vi "CIMAQ_ParticleFilter_MinMax.vi"(8 "error in (no error)":errorcluster, 9 "Max/Min":enum16{"Max", "Min"}(ring), 10 "Measurement Parameter":T1=35 items=["Center of Mass X", "Center of Mass Y", "First Pixel X", "First Pixel Y", "Bounding Rect Left", "Bounding Rect Top", "Bounding Rect Right", "Bounding Rect Bottom", "Max Feret Diameter Start X", "Max Feret Diameter Start Y", "Max Feret Diameter End X", "Max Feret Diameter End Y", "Max Horiz. Segment Length Left", "Max Horiz. Segment Length Right", "Max Horiz. Segment Length Row", "-", "Bounding Rect Width", "Bounding Rect Height", "Bounding Rect Diagonal", "Perimeter", "Convex Hull Perimeter", "Holes' Perimeter", "Max Feret Diameter", "Equivalent Ellipse Major Axis", "Equivalent Ellipse Minor Axis", "Equivalent Ellipse Minor Axis (Feret)", "Equivalent Rect Long Side", "Equivalent Rect Short Side", "Equivalent Rect Diagonal", "Equivalent Rect Short Side (Feret)", "Average Horiz. Segment Length", "Average Vert. Segment Length", "Hydraulic Radius", "Waddel Disk Diameter", "-", "Area", "Holes' Area", "Particle & Holes' Area", "Convex Hull Area", "Image Area", "-", "Number of Holes", "Number of Horiz. Segments", "Number of Vert. Segments", "-", "Orientation", "Max Feret Diameter Orientation", "-", "% Area/Image Area", "% Area/(Particle & Holes' Area)", "Ratio of Equivalent Ellipse Axes", "Ratio of Equivalent Rect Sides", "-", "Elongation Factor", "Compactness Factor", "Heywood Circularity Factor", "Type Factor", "-", "Sum X", "Sum Y", "Sum XX", "Sum XY", "Sum YY", "Sum XXX", "Sum XXY", "Sum XYY", "Sum YYY", "-", "Moment of Inertia XX", "Moment of Inertia XY", "Moment of Inertia YY", "Moment of Inertia XXX", "Moment of Inertia XXY", "Moment of Inertia XYY", "Moment of Inertia YYY", "Norm. Moment of Inertia XX", "Norm. Moment of Inertia XY", "Norm. Moment of Inertia YY", "Norm. Moment of Inertia XXX", "Norm. Moment of Inertia XXY", "Norm. Moment of Inertia XYY", "Norm. Moment of Inertia YYY", "Hu Moment 1", "Hu Moment 2", "Hu Moment 3", "Hu Moment 4", "Hu Moment 5", "Hu Moment 6", "Hu Moment 7"], 11 "Img":T2) -> (0 "error out":errorcluster, 3 "Img":T2)   [LabVIEW 2017]
uses:
  <vilib>/vision/Image Controls.llb/IMAQ Image.ctl
  <vilib>/vision/NI_Vision_Development_Module.lvlib
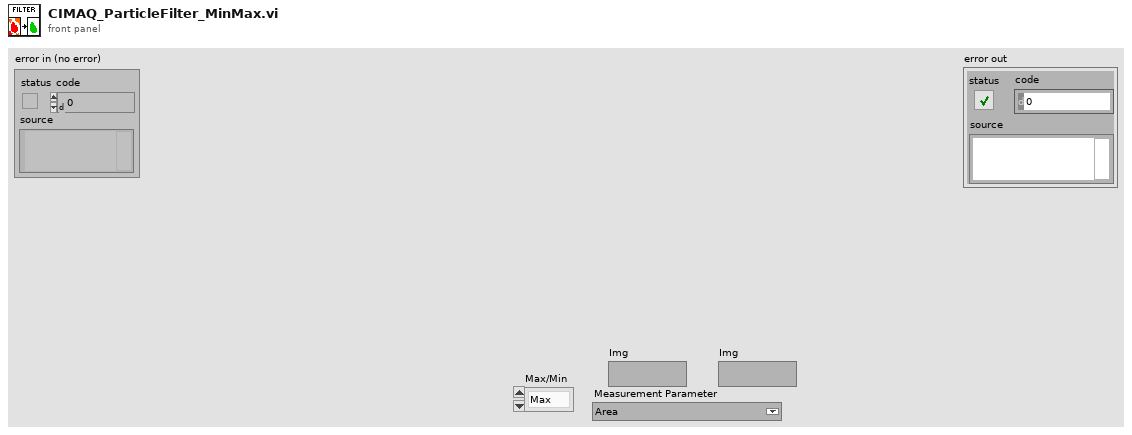
[diagram p1: front panel]
types:
  T1 = typedef "Particle Parameters" = i32
  T2 = typedef "IMAQ Image.ctl" = refnum<image>
  T3 = cluster{"Measurement Parameter":T1, "Range Lower Value":dbl, "Range Upper Value":dbl, "Range":bool, "Measurement Type":bool}
  T4 = cluster{"Measurement Parameter":T1, "Range Lower Value":dbl, "Range Upper Value":dbl, "Range":bool, "Measurement Type":bool}[]
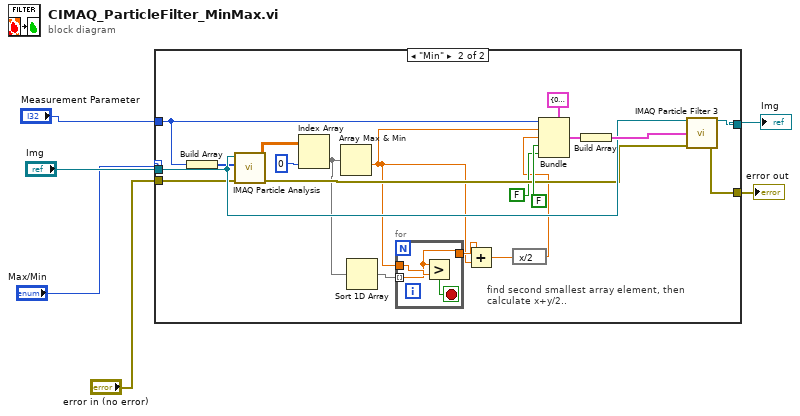
[diagram p0: block diagram]
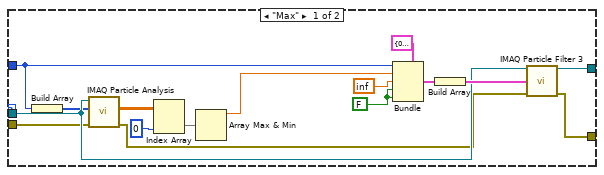
[diagram p2: hidden frame]
diagram:
  n1 = case shown="\"Min\"" "Max/Min" {
    tunnel: [w16 w38] -> w6
    tunnel: "Img" -> [w15 w37]
    tunnel: "Measurement Parameter" -> [w10 w33]
    tunnel: "error in (no error)" -> [w9 w32]
    tunnel: [w7 w30] -> w1
    frame "Max" {
      w20 = FALSE ("Range")
      n2 = Build Array(w10) -> (w11:T1[])
      n3 = call "IMAQ Particle Analysis"("error in (no error)"=w9, "Pixel Measurements"=w11, "Image"=w15) -> ("error out"=w8:errorcluster, "Particle Measurements (Pixels)"=w12:dbl[][])  [unwired: 3 in, 4 out]
      n4 = Index Array(array=w12, index (col)=0 ("disabled index (col)")) -> (element=w14:dbl[])  [unwired: 1 in]
      n5 = Array Max & Min(array=w14) -> (max value=w18:dbl)  [unwired: 3 out]
      n6 = Bundle(cluster=T3 {"Measurement Parameter"=0, "Range Lower Value"=0.0, "Range Upper Value"=0.0, "Range"=FALSE, "Measurement Type"=FALSE} ("Selection Value"), "Measurement Parameter"=w10, "Range Lower Value"=w18, "Range Upper Value"=inf, "Range"=w20, "Measurement Type"=w20) -> (w21:T3)
      n7 = Build Array(w21) -> (w22:T4)
      n8 = call "IMAQ Particle Filter 3"("Image Src"=w15, "Selection Values"=w22, "error in (no error)"=w8) -> ("Image Dst Out"=w16:T2, "error out"=w7:errorcluster)  [unwired: 10 in, 1 out]
    }
    frame "Min" {
      # "find second smallest array element, then\ncalculate x+y/2.."
      n9 = Build Array(w33) -> (w34:T1[])
      n10 = call "IMAQ Particle Analysis"("error in (no error)"=w32, "Pixel Measurements"=w34, "Image"=w37) -> ("error out"=w31:errorcluster, "Particle Measurements (Pixels)"=w35:dbl[][])  [unwired: 3 in, 4 out]
      n11 = Index Array(array=w35, index (col)=0 ("disabled index (col)")) -> (element=w28:dbl[])  [unwired: 1 in]
      n12 = Array Max & Min(array=w28) -> (min value=w25:dbl)  [unwired: 3 out]
      n13 = Sort 1D Array(array=w28) -> (sorted array=w27:dbl[])
      n14 = for {
        tunnel: w27 -> [w43] mode=indexing
        tunnel: w25 -> [w45]
        tunnel: [w43] -> w26
        stop <- w44 stop-if-true
        n15 = Greater?(x=w43, y=w45) -> (0:w44:bool)
      }
      n16 = Add(x=w26, y=w25) -> (x+y=w24:dbl)
      n17 = expression code="x/2"(w24) -> (w23:dbl)
      n18 = Bundle(cluster=T3 {"Measurement Parameter"=0, "Range Lower Value"=0.0, "Range Upper Value"=0.0, "Range"=FALSE, "Measurement Type"=FALSE} ("Selection Value"), "Measurement Parameter"=w33, "Range Lower Value"=w25, "Range Upper Value"=w23, "Range"=FALSE, "Measurement Type"=FALSE ("Range")) -> (w41:T3)
      n19 = Build Array(w41) -> (w42:T4)
      n20 = call "IMAQ Particle Filter 3"("Image Src"=w37, "Selection Values"=w42, "error in (no error)"=w31) -> ("Image Dst Out"=w38:T2, "error out"=w30:errorcluster)  [unwired: 10 in, 1 out]
    }
  }
  "Img" <- w6
  "error out" <- w1
